vi "Teleop.vi"(10 "Match Info":T1={"Autonomous Elapsed Seconds"=0.0, "TeleOp Elapsed Seconds"=0.0, "Disabled Elapsed Seconds"=0.0, "Visited Autonomous"=FALSE, "Visited TeleOp"=FALSE, "Visited Disabled"=FALSE, "Autonomous Settings"={"Autonomous Style"=enum."Independent", "VI Refnum"=refnum}}, 11 "Call Context":T2) -> ()   [LabVIEW 2014]
doc: "This VI is called for each TeleOp packet received from the DS where the robot is not disabled. It is often used to read from the joysticks and update I/O or to update setpoints for timed control loops. It should complete and return within 20 milliseconds or it may miss DS packets."
uses:
  <vilib>/Rock Robotics/WPI/DriverStation/WPI_DriverStationDerivedRobotMode.ctl
  <vilib>/Rock Robotics/WPI/DriverStation/WPI_DriverStationMatch Info.ctl
  <vilib>/Rock Robotics/WPI/RobotDrive/WPI_RobotDriveGetSetRefNum.vi
  <vilib>/Rock Robotics/WPI/Joystick/WPI_JoystickGetSetRefNum.vi
  <vilib>/Rock Robotics/Network Tables/SD Write Boolean Array.vi
  <vilib>/Rock Robotics/Network Tables/SD Write Numeric Array.vi
  <vilib>/Rock Robotics/Network Tables/SD Read Boolean.vi
  <vilib>/Rock Robotics/Network Tables/SD Read Number.vi
panel:
  out "limit switches":bool
  out "loop trigger":bool
  out "Button":dbl
  out "Limit Switch":dbl
  out "Sample Slider 0":dbl(slide) scale=0.0..5.0
  out "Sample Boolean 1":bool
  out "Sample Boolean 0":bool
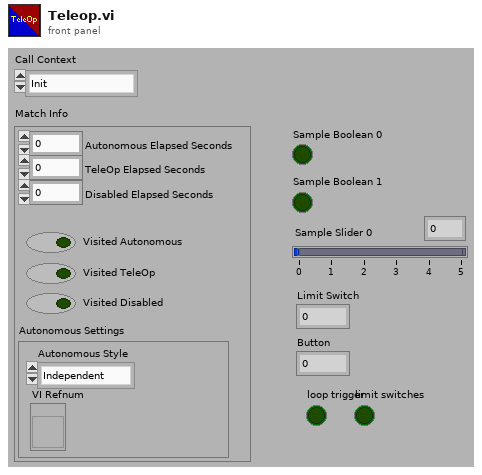
[diagram p1: front panel]
types:
  T1 = typedef "WPI_DriverStationMatch Info.ctl" = cluster{"Autonomous Elapsed Seconds":dbl, "TeleOp Elapsed Seconds":dbl, "Disabled Elapsed Seconds":dbl, "Visited Autonomous":bool, "Visited TeleOp":bool, "Visited Disabled":bool, "Autonomous Settings":cluster{"Autonomous Style":enum16{"Iterative", "Independent"}, "VI Refnum":refnum<vi>}}
  T2 = typedef "WPI_DriverStationDerivedRobotMode.ctl" = enum16{"Init", "Execute", "Stop"}
  T3 = typedef "WPI_RobotDriveDevRef.ctl" = cluster{"DevStatus":errorcluster, "Motors[]":T4[], "Square Inputs":bool, "Max Output":dbl}
  T4 = typedef "WPI_MotorControlDeviceRef.ctl" = cluster{"DeviceStatus":errorcluster, "Type":T5, "PWM":cluster{"Controller":T6, "PWM Channel":T7, "DeadBand":T8}, "CAN":cluster{"Device Number":u8, "Control Mode":T9, "Semaphore":T10, "Max Vout":dbl, "TalonSRX Control Mode":T11}, "Invert":bool, "TransformRef":T12, "InvTransformRef":T12}
  T5 = typedef "WPI_MotorControlType.ctl" = enum16{"PWM", "CAN", "CANTalonSRX"}
  T6 = typedef "FPGA_TypedefDigitalModule.ctl" = enum16{"Controller 1"}
  T7 = typedef "FPGA_DIOPWMChannel.ctl" = enum8{"PWM 0", "PWM 1", "PWM 2", "PWM 3", "PWM 4", "PWM 5", "PWM 6", "PWM 7", "PWM 8", "PWM 9", "PWM MXP 0", "PWM MXP 1", "PWM MXP 2", "PWM MXP 3", "PWM MXP 4", "PWM MXP 5", "PWM MXP 6", "PWM MXP 7", "PWM MXP 8", "PWM MXP 9", "Invalid"}
  T8 = typedef "WPI_PWMDeadband.ctl" = cluster{"Name":string, "maxPositivePwm":i32, "minPositivePwm":i32, "centerPwm":i32, "maxNegativePwm":i32, "minNegativePwm":i32, "angularRange":u16}
  T9 = typedef "WPI_CANJaguar_ControlMode.ctl" = enum8{"Percent VBus", "Current", "Speed", "Position", "Voltage"}
  T10 = typedef "Semaphore RefNum" = refnum<k1>
  T11 = typedef "WPI_CANTalonSRX_APIControlMode.ctl" = enum8{"Percent VBus", "Speed", "Position", "Slave", "Unchanged / Invalid"}
  T12 = typedef "WPI_PWMTransform_ConPane.ctl" = refnum<vi>
  T13 = typedef "WPI_JoystickDevRef.ctl" = cluster{"Device":T14}
  T14 = typedef "WPI_JoystickDeviceEnum.ctl" = enum16{"USB 0", "USB 1", "USB 2", "USB 3", "USB 4", "USB 5"}
  T15 = cluster{"Axes[0]":dbl, "Axes[1]":dbl, "Axes[2]":dbl, "Axes[3]":dbl, "Axes[4]":dbl, "Axes[5]":dbl, "Axes[6]":dbl, "Axes[7]":dbl, "Axes[8]":dbl}
  T16 = typedef "WPI_DigitalInputDevRef.ctl" = cluster{"DevStatus":errorcluster, "DIO Channel":T17, "Controller":T6}
  T17 = typedef "FPGA_DIOChannel.ctl" = enum8{"DIO 0", "DIO 1", "DIO 2", "DIO 3", "DIO 4", "DIO 5", "DIO 6", "DIO 7", "DIO 8", "DIO 9", "DIO MXP 0", "DIO MXP 1", "DIO MXP 2", "DIO MXP 3", "DIO MXP 4", "DIO MXP 5", "DIO MXP 6", "DIO MXP 7", "DIO MXP 8", "DIO MXP 9", "DIO MXP 10", "DIO MXP 11", "DIO MXP 12", "DIO MXP 13", "DIO MXP 14", "DIO MXP 15", "Invalid"}
  T18 = cluster{"Buttons[0]":bool, "Buttons[1]":bool, "Buttons[2]":bool, "Buttons[3]":bool, "Buttons[4]":bool, "Buttons[5]":bool, "Buttons[6]":bool, "Buttons[7]":bool, "Buttons[8]":bool}
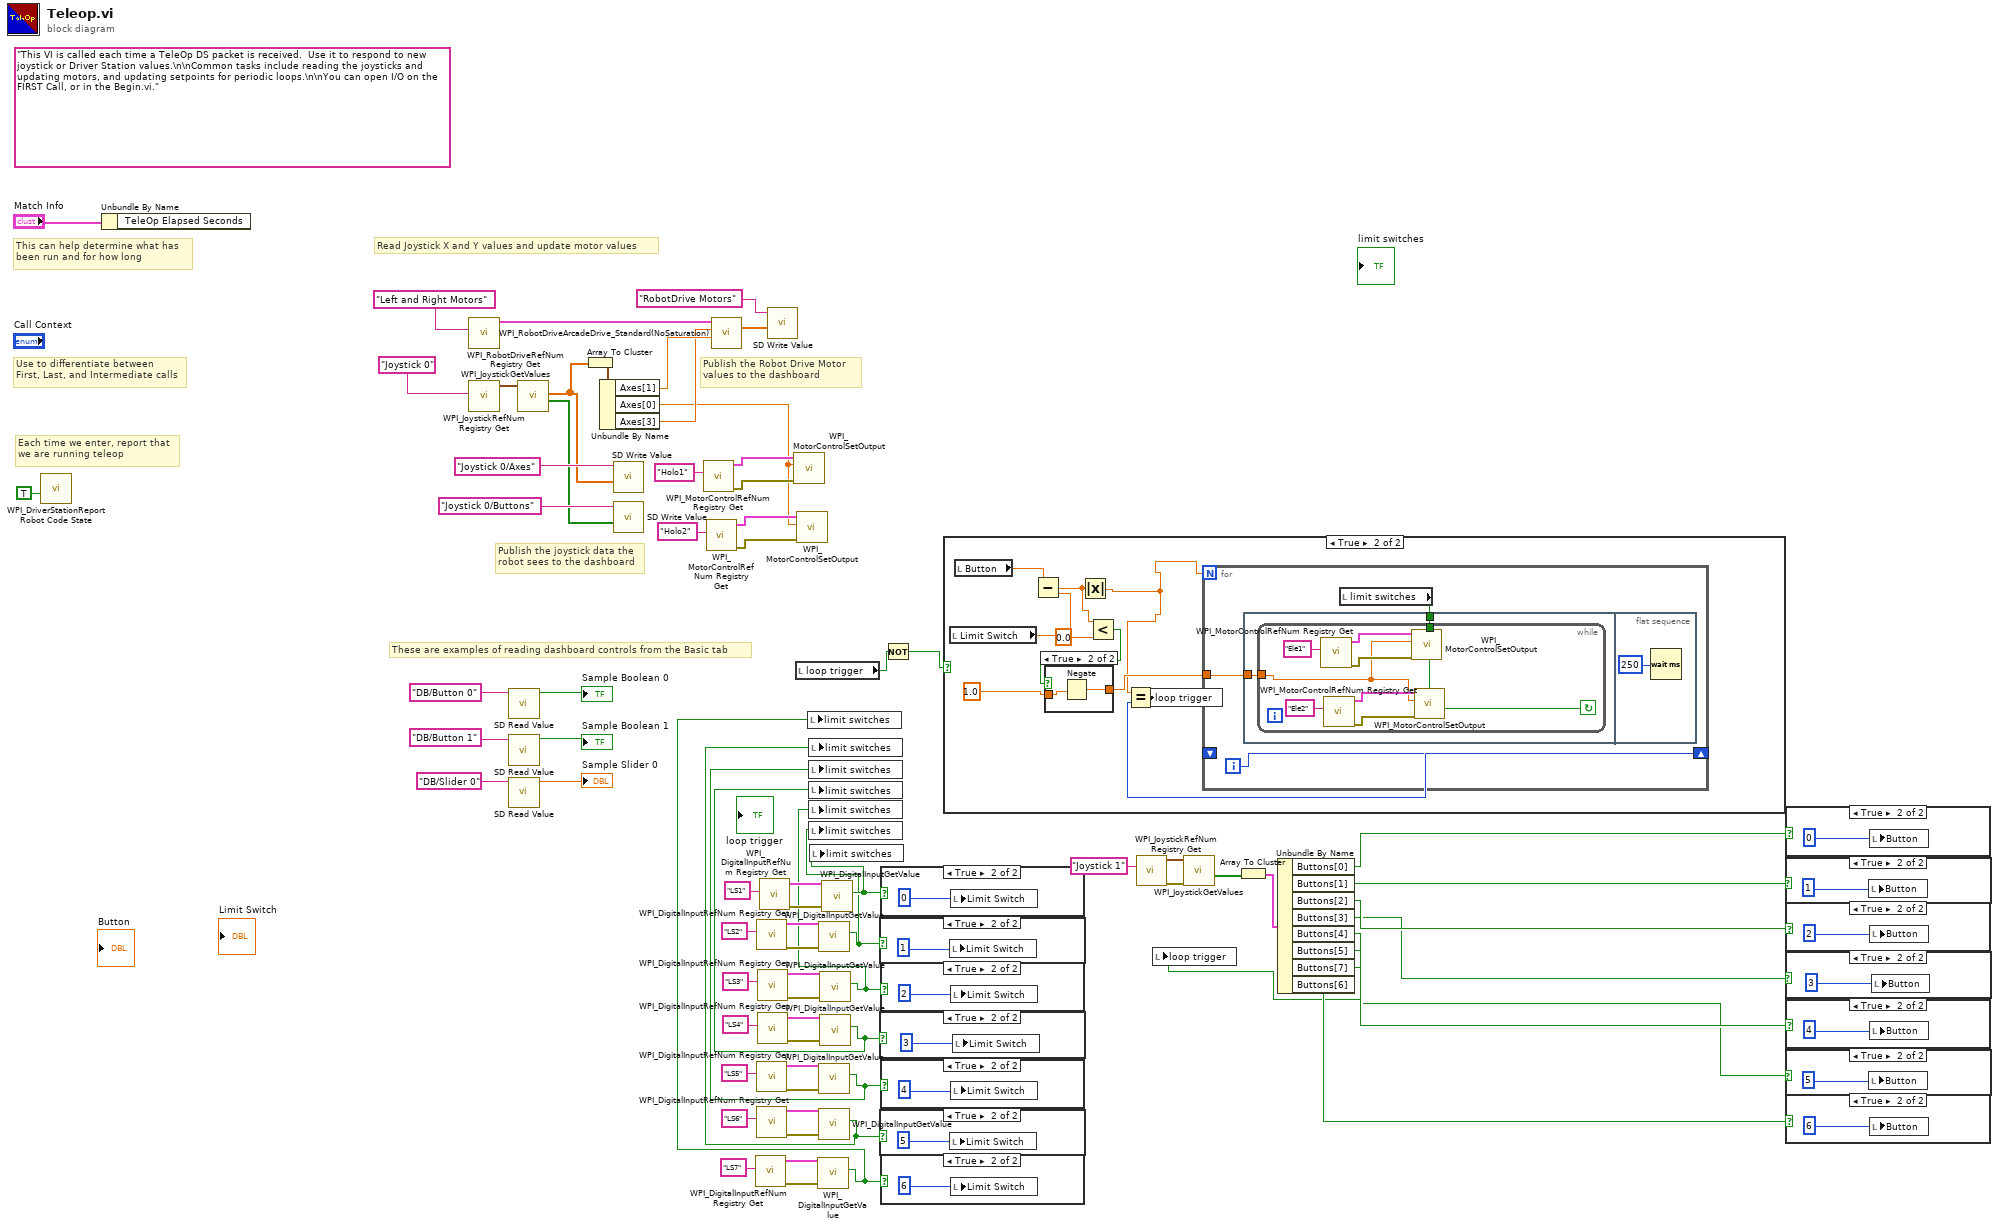
[diagram p0: block diagram]
diagram:
  (unwired) "This VI is called each time a TeleOp DS packet is received.  Use it to respond to new joystick or Driver Station values.\n\nCommon tasks include reading the joysticks and updating motors, and updating setpoints for periodic loops.\n\nYou can open I/O on the FIRST Call, or in the Begin.vi."
  # "These are examples of reading dashboard controls from the Basic tab"
  # "Publish the Robot Drive Motor\nvalues to the dashboard"
  # "Publish the joystick data the\nrobot sees to the dashboard"
  # "Each time we enter, report that\nwe are running teleop"
  # "Use to differentiate between\nFirst, Last, and Intermediate calls"
  # "This can help determine what has\nbeen run and for how long"
  # "Read Joystick X and Y values and update motor values"
  n1 = call <vilib>:"WPI_DriverStationReport Robot Code State.vi"("TeleOp"=TRUE ("Autonomous")) -> ()  [unwired: 10 in, 1 out]
  n2 = Unbundle By Name("Match Info") -> ()  [unwired: 1 out]
  n3 = call <vilib>:"WPI_RobotDriveRefNum Registry Get.vi"("refnum name"="Left and Right Motors") -> ("RobotDriveDevRef"=w69:T3)  [unwired: 1 in, 9 out]
  n4 = call <vilib>:"WPI_JoystickRefNum Registry Get.vi"("refnum name"="Joystick 0") -> ("JoystickDevRef"=w67:T13)  [unwired: 1 in, 9 out]
  n5 = call-poly <vilib>:"SD Read Value.vi"("Name"="DB/Button 0" ("refnum name")) -> ("Boolean"=→"Sample Boolean 0":bool)  [unwired: 8 in, 2 out]
  n6 = call-poly <vilib>:"SD Read Value.vi"("Name"="DB/Button 1" ("refnum name")) -> ("Boolean"=→"Sample Boolean 1":bool)  [unwired: 8 in, 2 out]
  n7 = call-poly <vilib>:"SD Read Value.vi"("Name"="DB/Slider 0" ("refnum name")) -> ("Numeric"=→"Sample Slider 0":dbl)  [unwired: 8 in, 2 out]
  n8 = call <vilib>:"WPI_JoystickGetValues.vi"("JoystickDevRef"=w67) -> ("Buttons"=w55:bool[], "Axes"=w54:dbl[])  [unwired: 6 in, 3 out]
  n9 = Array To Cluster(array=w54) -> (cluster=w53:T15)
  n10 = Unbundle By Name(w53) -> ("Axes[1]"=w52:dbl, "Axes[0]"=w44:dbl, "Axes[3]"=w45:dbl)
  n11 = call-poly <vilib>:"SD Write Value.vi"("Numeric Array"=w54, "Name"="Joystick 0/Axes") -> ()  [unwired: 8 in, 2 out]
  n12 = call-poly <vilib>:"SD Write Value.vi"("Boolean Array"=w55, "Name"="Joystick 0/Buttons") -> ()  [unwired: 8 in, 2 out]
  n13 = call <vilib>:"WPI_MotorControlRefNum Registry Get.vi"("refnum name"="Holo1") -> ("error out"=w50:errorcluster, "MotorControlDevRef"=w51:T4)  [unwired: 9 in]
  n14 = call <vilib>:"WPI_MotorControlRefNum Registry Get.vi"("refnum name"="Holo2") -> ("error out"=w47:errorcluster, "MotorControlDevRef"=w48:T4)  [unwired: 9 in]
  n15 = call <vilib>:"WPI_RobotDriveArcadeDrive_Standard(NoSaturation).vi"("Y axis value"=w52, "X axis value"=w45, "RobotDriveDevRef"=w69) -> ("Motor Values"=w58:dbl[])  [unwired: 1 in, 7 out]
  n16 = call <vilib>:"WPI_DigitalInputRefNum Registry Get.vi"("refnum name"="LS7") -> ("error out"=w23:errorcluster, "DigitalInputDevRef"=w24:T16)  [unwired: 9 in]
  n17 = call <vilib>:"WPI_DigitalInputRefNum Registry Get.vi"("refnum name"="LS2") -> ("error out"=w38:errorcluster, "DigitalInputDevRef"=w39:T16)  [unwired: 9 in]
  n18 = call <vilib>:"WPI_DigitalInputRefNum Registry Get.vi"("refnum name"="LS5") -> ("error out"=w29:errorcluster, "DigitalInputDevRef"=w30:T16)  [unwired: 9 in]
  n19 = call <vilib>:"WPI_DigitalInputRefNum Registry Get.vi"("refnum name"="LS6") -> ("error out"=w26:errorcluster, "DigitalInputDevRef"=w27:T16)  [unwired: 9 in]
  n20 = call <vilib>:"WPI_DigitalInputRefNum Registry Get.vi"("refnum name"="LS3") -> ("error out"=w35:errorcluster, "DigitalInputDevRef"=w36:T16)  [unwired: 9 in]
  n21 = call <vilib>:"WPI_DigitalInputRefNum Registry Get.vi"("refnum name"="LS4") -> ("error out"=w32:errorcluster, "DigitalInputDevRef"=w33:T16)  [unwired: 9 in]
  n22 = call <vilib>:"WPI_DigitalInputRefNum Registry Get.vi"("refnum name"="LS1") -> ("error out"=w41:errorcluster, "DigitalInputDevRef"=w42:T16)  [unwired: 9 in]
  n23 = call-poly <vilib>:"SD Write Value.vi"("Numeric Array"=w58, "Name"="RobotDrive Motors") -> ()  [unwired: 8 in, 2 out]
  n24 = call <vilib>:"WPI_MotorControlSetOutput.vi"("error in (no error)"=w50, "Output"=w44, "MotorControlDevRef"=w51) -> ()  [unwired: 6 in, 3 out]
  n25 = local read "loop trigger"() -> (w2:bool)
  n26 = call <vilib>:"WPI_MotorControlSetOutput.vi"("error in (no error)"=w47, "Output"=w44, "MotorControlDevRef"=w48) -> ()  [unwired: 6 in, 3 out]
  n27 = call <vilib>:"WPI_DigitalInputGetValue.vi"("error in (no error)"=w23, "DigitalInputDevRef"=w24) -> ("Value"=w3:bool)  [unwired: 7 in, 2 out]
  n28 = local write "limit switches"(w3) -> ()
  n29 = call <vilib>:"WPI_DigitalInputGetValue.vi"("error in (no error)"=w38, "DigitalInputDevRef"=w39) -> ("Value"=w8:bool)  [unwired: 7 in, 2 out]
  n30 = local write "limit switches"(w8) -> ()
  n31 = call <vilib>:"WPI_DigitalInputGetValue.vi"("error in (no error)"=w29, "DigitalInputDevRef"=w30) -> ("Value"=w5:bool)  [unwired: 7 in, 2 out]
  n32 = local write "limit switches"(w5) -> ()
  n33 = call <vilib>:"WPI_DigitalInputGetValue.vi"("error in (no error)"=w26, "DigitalInputDevRef"=w27) -> ("Value"=w4:bool)  [unwired: 7 in, 2 out]
  n34 = local write "limit switches"(w4) -> ()
  n35 = call <vilib>:"WPI_DigitalInputGetValue.vi"("error in (no error)"=w35, "DigitalInputDevRef"=w36) -> ("Value"=w7:bool)  [unwired: 7 in, 2 out]
  n36 = local write "limit switches"(w7) -> ()
  n37 = call <vilib>:"WPI_DigitalInputGetValue.vi"("error in (no error)"=w32, "DigitalInputDevRef"=w33) -> ("Value"=w6:bool)  [unwired: 7 in, 2 out]
  n38 = local write "limit switches"(w6) -> ()
  n39 = call <vilib>:"WPI_DigitalInputGetValue.vi"("error in (no error)"=w41, "DigitalInputDevRef"=w42) -> ("Value"=w9:bool)  [unwired: 7 in, 2 out]
  n40 = local write "limit switches"(w9) -> ()
  n41 = case shown="True" w8 {
    frame False {
    }
    frame True {
      n42 = local write "Limit Switch"(1) -> ()
    }
  }
  n43 = case shown="True" w6 {
    frame False {
    }
    frame True {
      n44 = local write "Limit Switch"(3) -> ()
    }
  }
  n45 = case shown="True" w4 {
    frame False {
    }
    frame True {
      n46 = local write "Limit Switch"(5) -> ()
    }
  }
  n47 = case shown="True" w9 {
    frame False {
    }
    frame True {
      n48 = local write "Limit Switch"(0) -> ()
    }
  }
  n49 = case shown="True" w7 {
    frame False {
    }
    frame True {
      n50 = local write "Limit Switch"(2) -> ()
    }
  }
  n51 = case shown="True" w5 {
    frame False {
    }
    frame True {
      n52 = local write "Limit Switch"(4) -> ()
    }
  }
  n53 = case shown="True" w3 {
    frame False {
    }
    frame True {
      n54 = local write "Limit Switch"(6) -> ()
    }
  }
  n55 = Not(x=w2) -> (.not. x?=w1:bool)
  n56 = case shown="True" w1 {
    frame False {
    }
    frame True {
      n57 = local read "Limit Switch"() -> (w87:dbl)
      n58 = local read "Button"() -> (w88:dbl)
      n59 = Subtract(x=w88, y=w87) -> (x-y=w83:dbl)
      n60 = Absolute Value(x=w83) -> (abs(x)=w79:dbl)
      n61 = Less?(x=w83, y=0.0) -> (x < y?=w82:bool)
      n62 = case shown="True" w82 {
        tunnel: 1.0 -> [w89 w91]
        tunnel: [w89 w90] -> w80
        frame False {
        }
        frame True {
          n63 = Negate(x=w91) -> (-x=w90:dbl)
        }
      }
      n64 = for {
        N: w79 -> [_]
        shift-right: [w94] -> w86
        shift-left: _ -> [_]
        tunnel: w80 -> [w92]
        i -> [w94]
        n65 = flat-sequence {
          tunnel: w93 -> [w96]
          tunnel: w92 -> [w95]
          frame #0 {
            n66 = while {
              tunnel: w96 -> [w104]
              tunnel: w95 -> [w97]
              stop <- w104 continue-if-true
              n67 = call <vilib>:"WPI_MotorControlRefNum Registry Get.vi"("refnum name"="Ele1") -> ("error out"=w102:errorcluster, "MotorControlDevRef"=w103:T4)  [unwired: 9 in]
              n68 = call <vilib>:"WPI_MotorControlRefNum Registry Get.vi"("refnum name"="Ele2") -> ("error out"=w99:errorcluster, "MotorControlDevRef"=w100:T4)  [unwired: 9 in]
              n69 = call <vilib>:"WPI_MotorControlSetOutput.vi"("error in (no error)"=w102, "Output"=w97, "MotorControlDevRef"=w103) -> ()  [unwired: 6 in, 3 out]
              n70 = call <vilib>:"WPI_MotorControlSetOutput.vi"("error in (no error)"=w99, "Output"=w97, "MotorControlDevRef"=w100) -> ()  [unwired: 6 in, 3 out]
            }
          }
          frame #1 {
            n71 = Wait (ms)(milliseconds to wait=u32 250) -> ()  [unwired: 1 out]
          }
        }
        n72 = local read "limit switches"() -> (w93:bool)
      }
      n73 = Equal?(x=w79, y=w86) -> (x = y?=w85:bool)
      n74 = local write "loop trigger"(w85) -> ()
    }
  }
  n75 = call <vilib>:"WPI_JoystickRefNum Registry Get.vi"("refnum name"="Joystick 1") -> ("error out"=w22:errorcluster, "JoystickDevRef"=w21:T13)  [unwired: 9 in]
  n76 = call <vilib>:"WPI_JoystickGetValues.vi"("error in (no error)"=w22, "JoystickDevRef"=w21) -> ("Buttons"=w20:bool[])  [unwired: 5 in, 4 out]
  n77 = Array To Cluster(array=w20) -> (cluster=w19:T18)
  n78 = Unbundle By Name(w19) -> ("Buttons[0]"=w18:bool, "Buttons[1]"=w17:bool, "Buttons[2]"=w16:bool, "Buttons[3]"=w15:bool, "Buttons[4]"=w14:bool, "Buttons[5]"=w13:bool, "Buttons[7]"=w10:bool, "Buttons[6]"=w12:bool)
  n79 = local write "loop trigger"(w10) -> ()
  n80 = case shown="True" w17 {
    frame False {
    }
    frame True {
      n81 = local write "Button"(1) -> ()
    }
  }
  n82 = case shown="True" w15 {
    frame False {
    }
    frame True {
      n83 = local write "Button"(3) -> ()
    }
  }
  n84 = case shown="True" w13 {
    frame False {
    }
    frame True {
      n85 = local write "Button"(5) -> ()
    }
  }
  n86 = case shown="True" w18 {
    frame False {
    }
    frame True {
      n87 = local write "Button"(0) -> ()
    }
  }
  n88 = case shown="True" w16 {
    frame False {
    }
    frame True {
      n89 = local write "Button"(2) -> ()
    }
  }
  n90 = case shown="True" w14 {
    frame False {
    }
    frame True {
      n91 = local write "Button"(4) -> ()
    }
  }
  n92 = case shown="True" w12 {
    frame False {
    }
    frame True {
      n93 = local write "Button"(6) -> ()
    }
  }
